vi "VI_UsingXNode.vi"(5 "input string":string) -> (2 "remaining string":string)   [LabVIEW 2012]
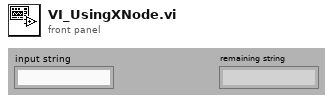
[diagram p1: front panel]
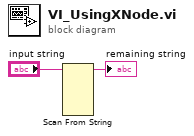
[diagram p0: block diagram]
diagram:
  n1 = Scan From String(input string="input string") -> (remaining string=→"remaining string":string)  [unwired: 9 in, 2 out]
